vi "SetMotors.vi"() -> ()   [LabVIEW 2018]
panel:
  in  "Motor 1":dbl
  in  "Motor 3":dbl
  in  "Motor 0":dbl
  in  "Motor 2":dbl
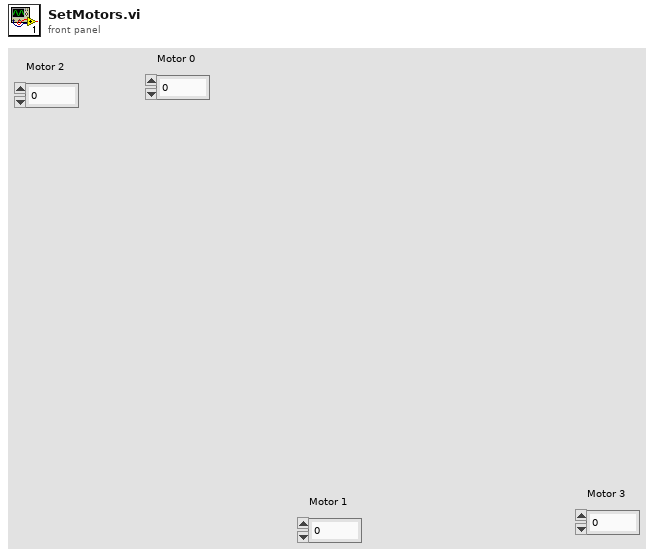
[diagram p1: front panel]
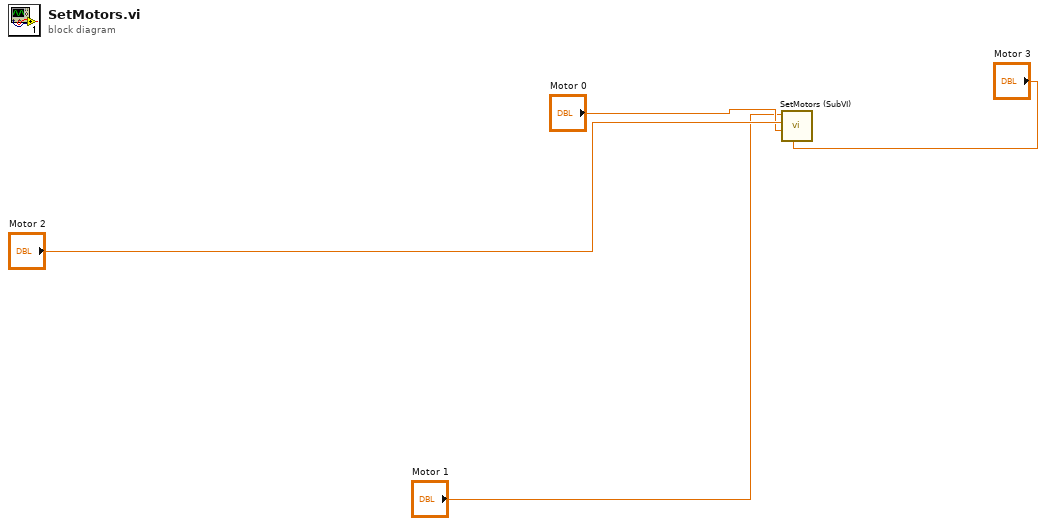
[diagram p0: block diagram]
diagram:
  n1 = call "SetMotors (SubVI).vi"("Oikea"="Motor 3", "Etu"="Motor 0", "Vasen"="Motor 2", "Taka"="Motor 1") -> ()  [unwired: 8 in]
